vi "Set_NeedleValve.vi"(11 "Numeric":i32) -> ()   [LabVIEW 2016]
uses:
  Monitors/Utility/Monitor Communication/S16/VTI-control.ctl
  Global Variables/Data_Display_global.vi
  Global Variables/global.vi
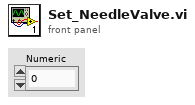
[diagram p1: front panel]
types:
  T1 = typedef "VTI-control.ctl" = cluster{"Set VTI SP":bool, "Change NV Status":bool, "Set NV Setpoint":bool, "Change Heater Status":bool, "Set Heater Setpoint":bool, "Setpoint (K)":dbl, "Rate (K/min)":dbl, "Setpoint Heater":dbl, "Setpoint NV":dbl, "Change Auto PID":bool, "Stop Sweep":bool}
  T2 = typedef "VTI-cluster.ctl" = cluster{"Temperatur (K)":dbl, "Setpoint (K)":dbl, "Rate (K/min)":dbl, "Heater (%)":dbl, "NV (%)":dbl, "Heater Manual":bool, "NV Manual":bool, "Go to Set":bool, "Pressure":dbl, "Heater SP":dbl, "Valid?":bool, "Set Heater SP":bool, "Set NV SP":bool, "Heater (%) Display":dbl, "NV (%) Display":dbl, "NV Setpoint":dbl, "Change Heater Status":bool, "Change NV Status":bool, "Sample 3":dbl, "Sample 2":dbl, "Sweep-State":bool, "Set Auto PID":bool, "Auto PID":bool, "Stopp":bool, "Setpoint-Sweep":dbl}
  T3 = typedef "VTI-status.ctl" = cluster{"Temperatur (K)":dbl, "Heater (%)":dbl, "NV (%)":dbl, "Heater Manual":bool, "NV Manual":bool, "Pressure":dbl, "Valid?":bool, "Heater (%) Display":dbl, "NV (%) Display":dbl, "Sample 2":dbl, "Sample 3":dbl, "Auto PID":bool, "Sweep-Status":bool, "Setpoint-Sweep":dbl}
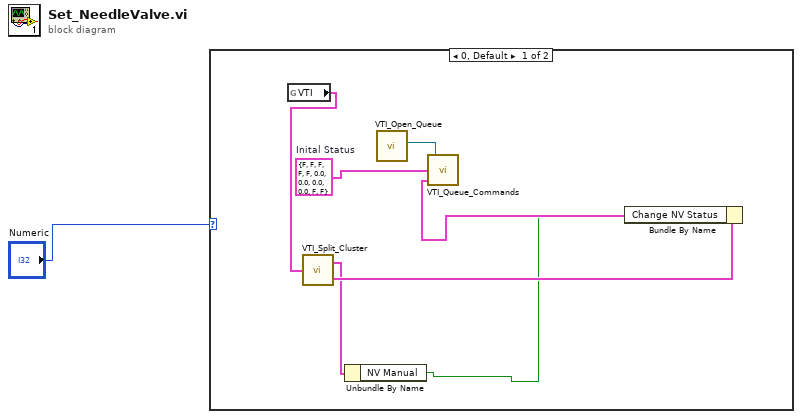
[diagram p0: block diagram]
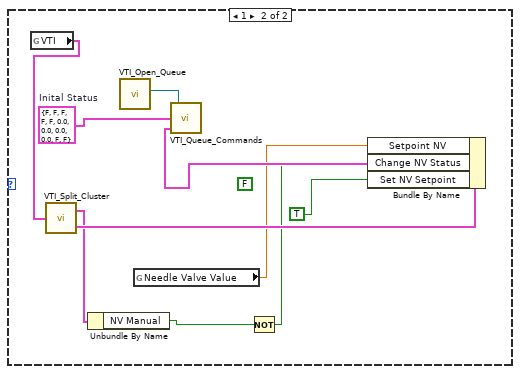
[diagram p2: hidden frame]
diagram:
  n1 = case shown="0, Default" "Numeric" {
    frame 0, Default {
      w7 = T1 {"Set VTI SP"=FALSE, "Change NV Status"=FALSE, "Set NV Setpoint"=FALSE, "Change Heater Status"=FALSE, "Set Heater Setpoint"=FALSE, "Setpoint (K)"=0.0, "Rate (K/min)"=0.0, "Setpoint Heater"=0.0, "Setpoint NV"=0.0, "Change Auto PID"=FALSE, "Stop Sweep"=FALSE}  # Inital Status
      n2 = global read "Data_Display_global.vi" "VTI"() -> (w6:T2)
      n3 = call "VTI_Split_Cluster.vi"("VTI"=w6) -> ("VTI Status"=w3:T3, "VTI Control"=w5:T1)
      n4 = Unbundle By Name(w3) -> ("NV Manual"=w2:bool)
      n5 = call "VTI_Open_Queue.vi"() -> ("queue out"=w8:refnum<queue>)  [unwired: 10 in, 1 out]
      n6 = Bundle By Name(cluster=w5, "Change NV Status"=w2) -> (w4:T1)
      n7 = call "VTI_Queue_Commands.vi"("VTI Control"=w4, "Last status"=w7, "20TVTI Queue"=w8) -> ()  [unwired: 1 out]
    }
    frame 1 {
      w17 = T1 {"Set VTI SP"=FALSE, "Change NV Status"=FALSE, "Set NV Setpoint"=FALSE, "Change Heater Status"=FALSE, "Set Heater Setpoint"=FALSE, "Setpoint (K)"=0.0, "Rate (K/min)"=0.0, "Setpoint Heater"=0.0, "Setpoint NV"=0.0, "Change Auto PID"=FALSE, "Stop Sweep"=FALSE}  # Inital Status
      (unwired) FALSE
      n8 = global read "Data_Display_global.vi" "VTI"() -> (w16:T2)
      n9 = call "VTI_Split_Cluster.vi"("VTI"=w16) -> ("VTI Status"=w11:T3, "VTI Control"=w15:T1)
      n10 = Unbundle By Name(w11) -> ("NV Manual"=w10:bool)
      n11 = call "VTI_Open_Queue.vi"() -> ("queue out"=w18:refnum<queue>)  [unwired: 10 in, 1 out]
      n12 = global read "global.vi" "Needle Valve Value"() -> (w13:dbl)
      n13 = Not(x=w10) -> (.not. x?=w9:bool)
      n14 = Bundle By Name(cluster=w15, "Setpoint NV"=w13, "Change NV Status"=w9, "Set NV Setpoint"=TRUE) -> (w14:T1)
      n15 = call "VTI_Queue_Commands.vi"("VTI Control"=w14, "Last status"=w17, "20TVTI Queue"=w18) -> ()  [unwired: 1 out]
    }
  }
